vi "Arm_Graphic.vi"(10 "Boundary":T1={"X max"=310.0, "X min"=147.0, "Z max"=148.0, "Z min"=-92.0}, 11 "Calibrated Oculus Data":T2={"head"={"orientation"={"roll"=0.0, "pitch"=0.0, "yaw"=0.0}, "position"={"x"=0.0, "y"=0.0, "z"=0.0}}, "hands"={"left"={"position"={"x"=0.0, "y"=0.0, "z"=0.0}, "orientation"={"roll"=0.0, "pitch"=0.0, "yaw"=0.0}}, "right"={"position"={"x"=290.0, "y"=70.0, "z"=7.0}, "orientation"={"roll"=0.0, "pitch"=0.0, "yaw"=0.0}}}, "buttons"={"a"=FALSE, "b"=FALSE, "x"=FALSE, "y"=FALSE, "menu"=FALSE, "leftTrig"=0.0, "rightTrig"=0.0, "leftGrip"=0.0, "rightGrip"=0.0, "left_jstick"={"x"=0.0, "y"=0.0, "button"=FALSE}, "right_jstick"={"x"=0.0, "y"=0.0, "button"=FALSE}}}) -> (3 "Scene Display":refnum<vi>(3d-picture))   [LabVIEW 2017]
uses:
  Calibrated Oculus Data.ctl
  <vilib>/Utility/miscctls.llb/LVRectTypeDef.ctl
  <vilib>/picture/3D Picture Control/Object/Create Object (drawable).vi
  <vilib>/picture/3D Picture Control/Object/Create Object (name).vi
  <vilib>/picture/3D Picture Control/Object/Add Object (reference).vi
  <vilib>/express/express arith-compare/Formula/XNode/ExpressFormulaBlockNode.xnode
  <vilib>/picture/3D Picture Control/NI_3D Picture Control.lvlib
panel:
  in  "Axis label?":bool=TRUE
  out "Phi1":dbl=1.0525167643137534
  in  "R2":sgl=158.8
  in  "R1":sgl=142.0
  out "R3'":dbl=260.2363744396104
  out "r3 |x,y|":dbl=298.328677803526
  out "Theta1":sgl=1.0769706
  out "Omega":sgl=0.23684876
  in  "Up Direction":cluster{"X":sgl, "Y":sgl, "Z":sgl}={"X"=0.0, "Y"=1.0, "Z"=0.0}
  in  "Target":cluster{"X":sgl, "Y":sgl, "Z":sgl}={"X"=100.0, "Y"=100.0, "Z"=0.0}
  in  "Camera Position":cluster{"X":sgl, "Y":sgl, "Z":sgl}={"X"=300.0, "Y"=400.0, "Z"=400.0}
  in  "Rendering Destination":enum16{"Scene Window", "Scene Display"}(ring)=enum."Scene Display"
  in  "Camera Controller":enum16{"None", "Spherical", "Flying"}(ring)=enum."Spherical"
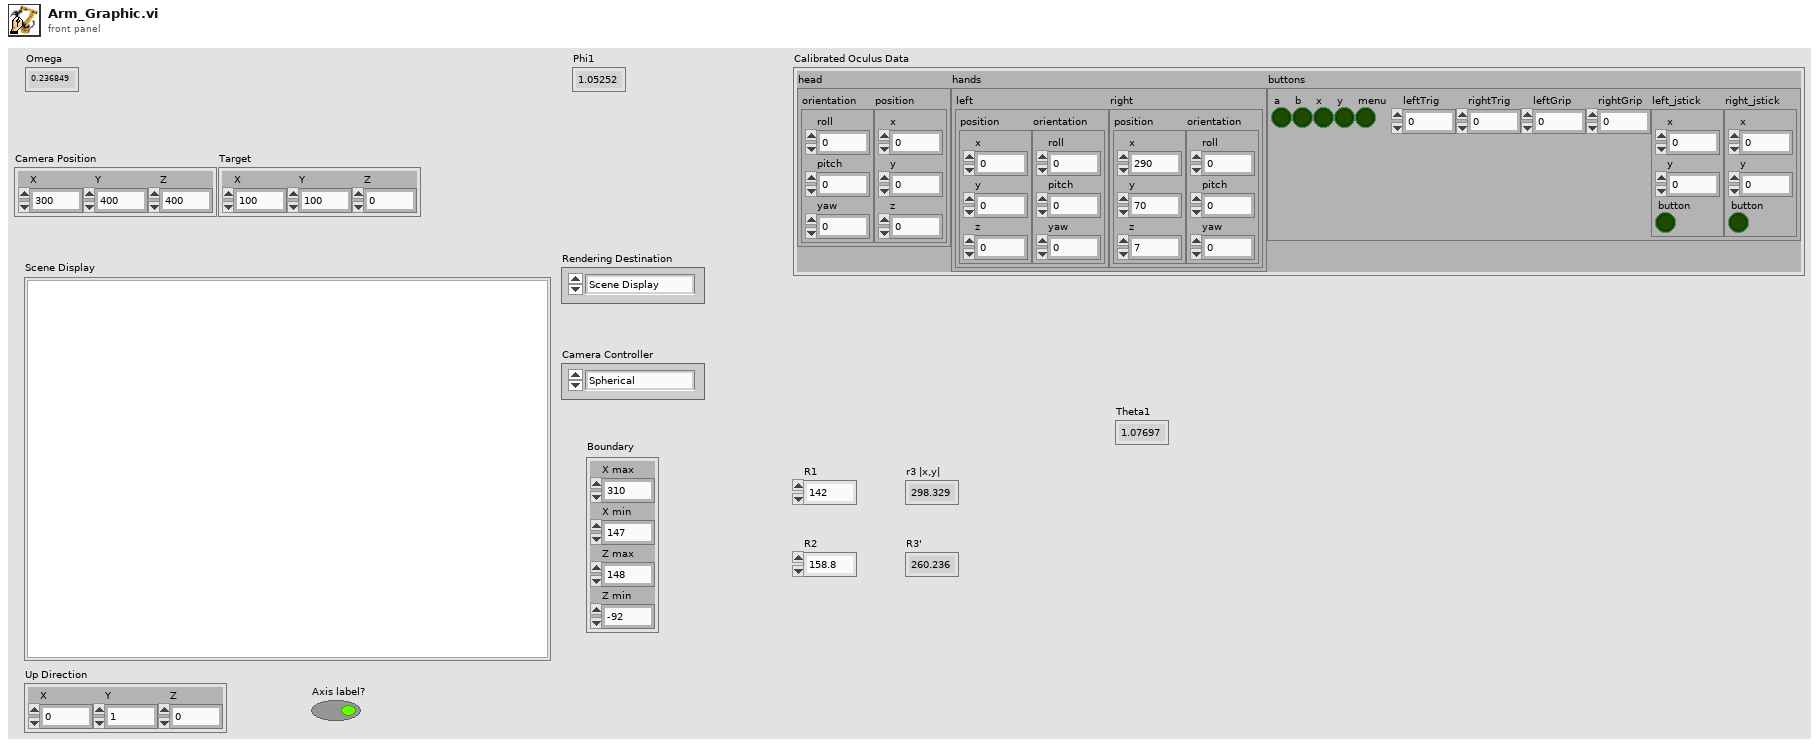
[diagram p1: front panel]
types:
  T1 = cluster{"X max":dbl, "X min":dbl, "Z max":dbl, "Z min":dbl}
  T2 = typedef "Calibrated Oculus Data.ctl" = cluster{"head":cluster{"orientation":cluster{"roll":dbl, "pitch":dbl, "yaw":dbl}, "position":cluster{"x":dbl, "y":dbl, "z":dbl}}, "hands":cluster{"left":cluster{"position":cluster{"x":dbl, "y":dbl, "z":dbl}, "orientation":cluster{"roll":dbl, "pitch":dbl, "yaw":dbl}}, "right":cluster{"position":cluster{"x":dbl, "y":dbl, "z":dbl}, "orientation":cluster{"roll":dbl, "pitch":dbl, "yaw":dbl}}}, "buttons":cluster{"a":bool, "b":bool, "x":bool, "y":bool, "menu":bool, "leftTrig":dbl, "rightTrig":dbl, "leftGrip":dbl, "rightGrip":dbl, "left_jstick":cluster{"x":dbl, "y":dbl, "button":bool}, "right_jstick":cluster{"x":dbl, "y":dbl, "button":bool}}}
  T3 = cluster{"Red":sgl, "Green":sgl, "Blue":sgl, "Alpha":sgl}
  T4 = cluster{"head":cluster{"orientation":cluster{"roll":dbl, "pitch":dbl, "yaw":dbl}, "position":cluster{"x":dbl, "y":dbl, "z":dbl}}, "hands":cluster{"left":cluster{"position":cluster{"x":dbl, "y":dbl, "z":dbl}, "orientation":cluster{"roll":dbl, "pitch":dbl, "yaw":dbl}}, "right":cluster{"position":cluster{"x":dbl, "y":dbl, "z":dbl}, "orientation":cluster{"roll":dbl, "pitch":dbl, "yaw":dbl}}}, "buttons":cluster{"a":bool, "b":bool, "x":bool, "y":bool, "menu":bool, "leftTrig":dbl, "rightTrig":dbl, "leftGrip":dbl, "rightGrip":dbl, "left_jstick":cluster{"x":dbl, "y":dbl, "button":bool}, "right_jstick":cluster{"x":dbl, "y":dbl, "button":bool}}}
  T5 = enum16{"Open", "Minimized", "Maximized", "Hidden"}
  T6 = typedef "LVRectTypeDef.ctl" = cluster{"Left":i16, "Top":i16, "Right":i16, "Bottom":i16}
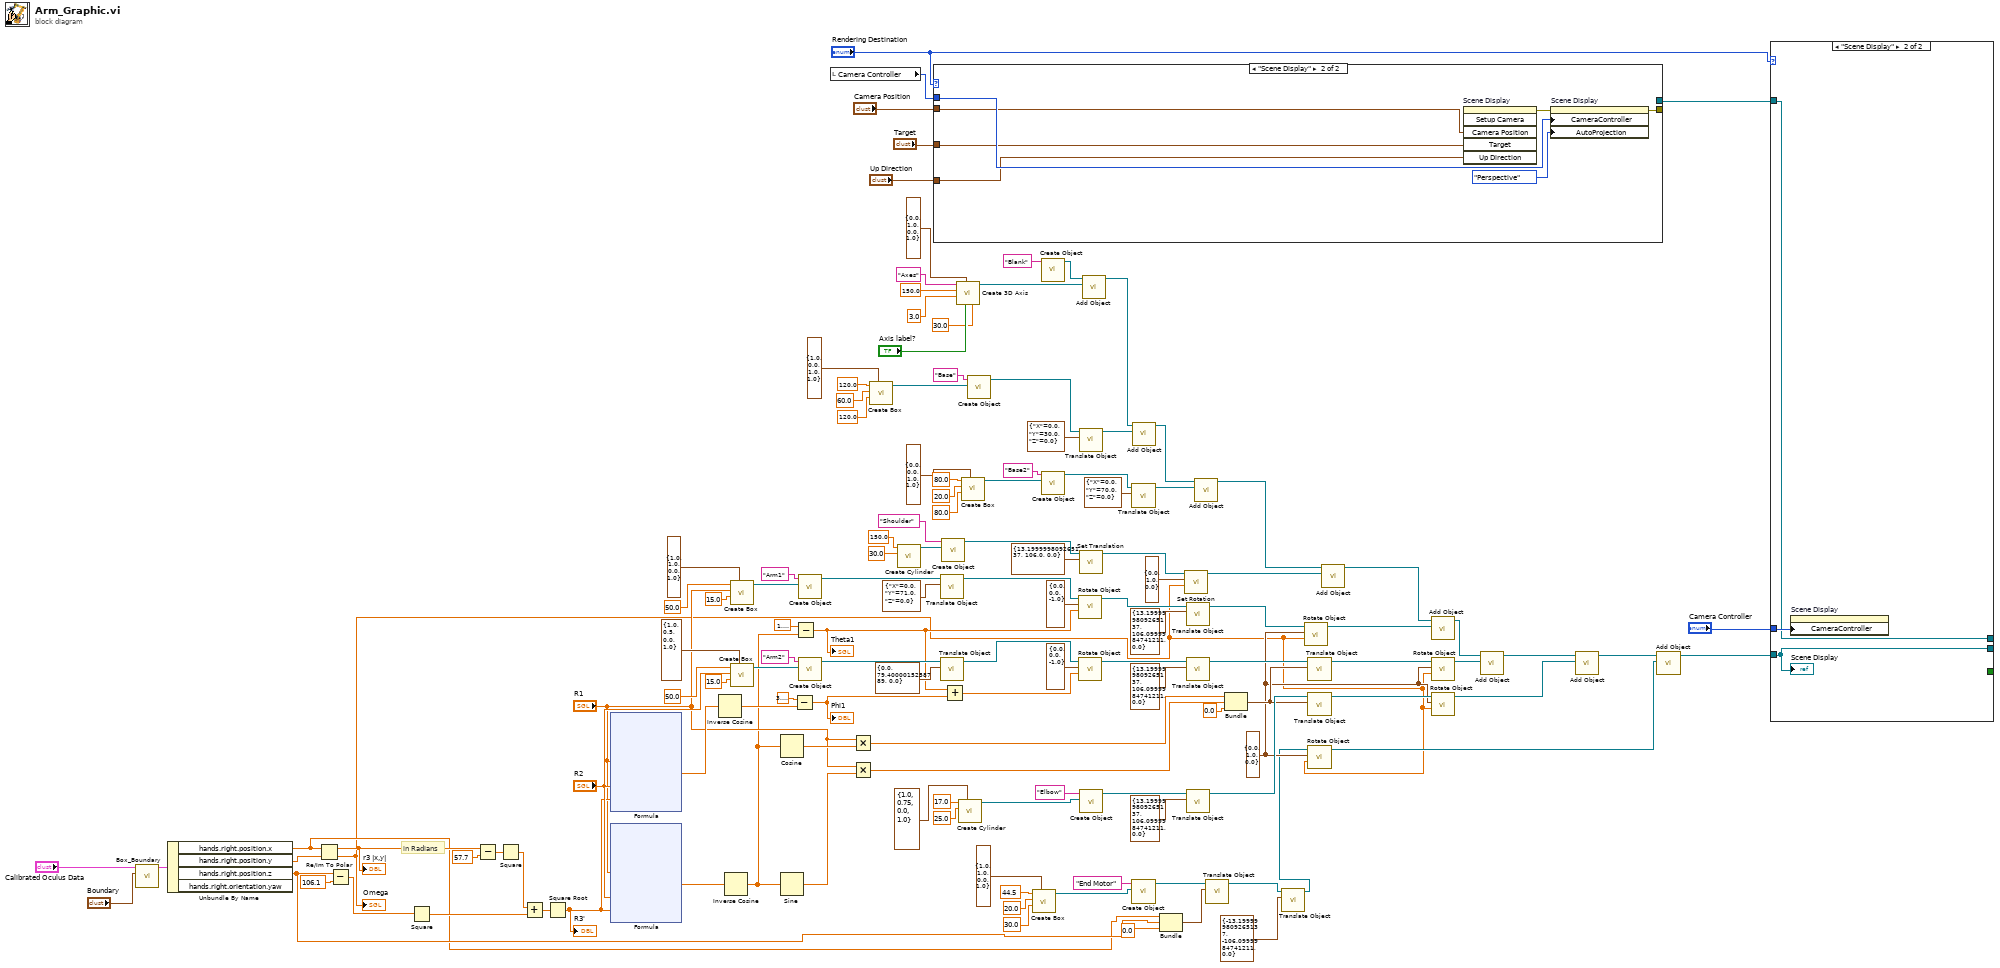
[diagram p0: block diagram]
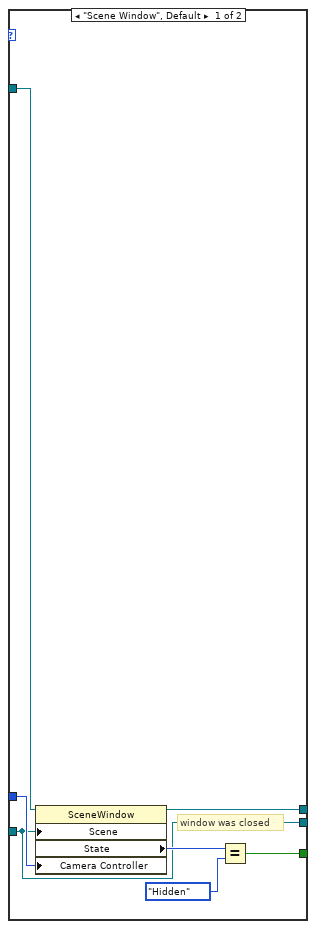
[diagram p2: hidden frame]
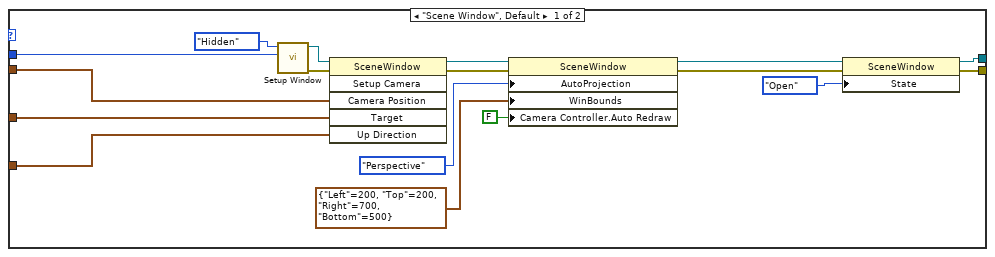
[diagram p3: hidden frame]
diagram:
  w9 = cluster{"X":sgl, "Y":sgl, "Z":sgl} {"X"=0.0, "Y"=1.0, "Z"=0.0} ("Axis")
  # "in Radians"
  n1 = call "Box_Boundary.vi"("Boundary"="Boundary", "Oculus Data in"="Calibrated Oculus Data") -> ("Oculus Data out"=w22:T4)  [unwired: 8 in, 1 out]
  n2 = Unbundle By Name(w22) -> ("hands.right.position.x"=w5:dbl, "hands.right.position.y"=w88:dbl, "hands.right.position.z"=w6:dbl)  [unwired: 1 out]
  n3 = Re/Im To Polar(2:w88, 3:w5) -> (0:w1:dbl, 1:w79:dbl)
  "Omega" <- w1
  "r3 |x,y|" <- w79
  n4 = Subtract(x=w6, y=106.1) -> (x-y=w76:dbl)
  n5 = Square(x=w76) -> (x^2=w74:dbl)
  n6 = Subtract(x=w79, y=57.7) -> (x-y=w77:dbl)
  n7 = Square(x=w77) -> (x^2=w75:dbl)
  n8 = Add(x=w75, y=w74) -> (x+y=w73:dbl)
  n9 = Square Root(x=w73) -> (sqrt(x)=w51:dbl)
  "R3'" <- w51
  n10 = xnode "Formula"("R1"="R1", "R2"="R2", "R3"=w51) -> ("Result"=w53:dbl)  [unwired: 1 in, 1 out]
  n11 = xnode "Formula"("R1"="R1", "R2"="R2", "R3"=w51) -> ("Result"=w72:dbl)  [unwired: 1 in, 1 out]
  n12 = Inverse Cosine(1:w53) -> (0:w49:dbl)
  n13 = Inverse Cosine(1:w72) -> (0:w37:dbl)
  n14 = call <vilib>:"Create Box.vi"("Color"=T3 {"Red"=1.0, "Green"=1.0, "Blue"=0.0, "Alpha"=1.0}, "Length Z"=sgl 15.0, "Length Y"="R1", "Length X"=sgl 50.0) -> ("New Box Refnum"=w133:refnum<vi>)  [unwired: 6 in, 1 out]
  n15 = call <vilib>:"Create Box.vi"("Color"=T3 {"Red"=1.0, "Green"=0.5, "Blue"=0.0, "Alpha"=1.0}, "Length Z"=sgl 15.0, "Length Y"="R2", "Length X"=sgl 50.0) -> ("New Box Refnum"=w101:refnum<vi>)  [unwired: 6 in, 1 out]
  n16 = Cosine(x=w37) -> (cos(x)=w40:dbl)
  n17 = Sine(x=w37) -> (sin(x)=w39:dbl)
  n18 = Subtract(x=3.141592653589793, y=w49) -> (x-y=w48:dbl)
  "Phi1" <- w48
  n19 = Subtract(x=1.5707963267948966, y=w37) -> (x-y=w47:dbl)
  "Theta1" <- w47
  n20 = call-poly <vilib>:"Create Object.vi"("Geometry"=w133, "Name"="Arm1") -> ("Scene:New Object"=w63:refnum<vi>)  [unwired: 8 in, 1 out]
  n21 = call-poly <vilib>:"Create Object.vi"("Geometry"=w101, "Name"="Arm2") -> ("Scene:New Object"=w55:refnum<vi>)  [unwired: 8 in, 1 out]
  n22 = local read "Camera Controller"() -> (w130:enum16{"None", "Spherical", "Flying"})
  n23 = Multiply(x="R1", y=w40) -> (x*y=w36:dbl)
  n24 = Multiply(x="R1", y=w39) -> (x*y=w35:dbl)
  n25 = call <vilib>:"Create Box.vi"("Color"=T3 {"Red"=1.0, "Green"=0.0, "Blue"=1.0, "Alpha"=1.0}, "Length Z"=sgl 120.0, "Length Y"=sgl 60.0, "Length X"=sgl 120.0) -> ("New Box Refnum"=w131:refnum<vi>)  [unwired: 6 in, 1 out]
  n26 = call <vilib>:"Create Cylinder.vi"("Radius"=sgl 30.0 ("Length Y"), "Height"=sgl 150.0 ("Length X")) -> ("New Cylinder Refnum"=w122:refnum<vi>)  [unwired: 8 in, 1 out]
  n27 = case shown="\"Scene Display\"" "Rendering Destination" {
    tunnel: w130 -> [w143 w157]
    tunnel: "Camera Position" -> [w145 w156]
    tunnel: "Target" -> [w146 w155]
    tunnel: "Up Direction" -> [w147 w154]
    tunnel: [w140 _] -> w87
    tunnel: [w136 w153] -> _
    frame "Scene Window", Default {
      n28 = call <vilib>:"Setup Window.vi"("Camera Controller"=w143, "Window State"=T5."Hidden") -> ("error out"=w139:errorcluster, "New Window Refnum"=w149:refnum<vi>)  [unwired: 1 in, 7 out]
      n29 = invoke class="SceneWindow" method="Setup Camera"(reference=w149, error in=w139, "Camera Position"=w145, "Target"=w146, "Up Direction"=w147) -> (reference out=w148:refnum<vi>, error out=w138:errorcluster)  [unwired: 1 in, 4 out]
      n30 = property class="SceneWindow"(reference=w148, error in=w138, "AutoProjection"=enum16{"None", "Perspective", "Orthographic"}."Perspective" ("Automatic Projection Mode"), "WinBounds"=T6 {"Left"=200, "Top"=200, "Right"=700, "Bottom"=500} ("Window Bounds"), "Camera Controller.Auto Redraw"=FALSE ("Camera Controller:Auto Redraw")) -> (reference out=w141:refnum<vi>, error out=w137:errorcluster)
      n31 = property class="SceneWindow"(reference=w141, error in=w137, "State"=T5."Open" ("Window State")) -> (reference out=w140:refnum<vi>, error out=w136:errorcluster)
    }
    frame "Scene Display" {
      n32 = invoke on="Scene Display" class="SceneGraphDisp (strict)" method="Setup Camera"("Camera Position"=w156, "Target"=w155, "Up Direction"=w154) -> (error out=w158:errorcluster)  [unwired: 3 in, 5 out]
      n33 = property on="Scene Display" class="SceneGraphDisp (strict)"(error in=w158, "CameraController"=w157, "AutoProjection"=enum16{"None", "Perspective", "Orthographic"}."Perspective" ("Auto Projection Mode")) -> (error out=w153:errorcluster)  [unwired: 1 in, 1 out]
    }
  }
  n34 = call <vilib>:"Translate Object.vi"("Translation"=cluster{"X":sgl, "Y":sgl, "Z":sgl} {"X"=0.0, "Y"=71.0, "Z"=0.0}, "Scene.Object In"=w63) -> ("Scene.Object Out"=w65:refnum<vi>)  [unwired: 1 in, 8 out]
  n35 = call <vilib>:"Translate Object.vi"("Translation"=cluster{"X":sgl, "Y":sgl, "Z":sgl} {"X"=0.0, "Y"=79.4, "Z"=0.0}, "Scene.Object In"=w55) -> ("Scene.Object Out"=w58:refnum<vi>)  [unwired: 1 in, 8 out]
  n36 = call-poly <vilib>:"Create Object.vi"("Geometry"=w122, "Name"="Shoulder") -> ("Scene:New Object"=w83:refnum<vi>)  [unwired: 8 in, 1 out]
  n37 = Add(x=w47, y=w48) -> (x+y=w46:dbl)
  n38 = call <vilib>:"Create 3D Axis.vi"("Character Size"=sgl 30.0, "Axis label?"="Axis label?", "Color"=T3 {"Red"=0.0, "Green"=1.0, "Blue"=0.0, "Alpha"=1.0}, "Radius"=sgl 3.0, "Length"=sgl 150.0, "Name"="Axes") -> ("New Object Refnum"=w97:refnum<vi>)  [unwired: 4 in, 1 out]
  n39 = call <vilib>:"Create Cylinder.vi"("Color"=T3 {"Red"=1.0, "Green"=0.75, "Blue"=0.0, "Alpha"=1.0}, "Radius"=sgl 25.0 ("Length Y"), "Height"=sgl 17.0 ("Length X")) -> ("New Cylinder Refnum"=w33:refnum<vi>)  [unwired: 7 in, 1 out]
  n40 = call <vilib>:"Create Box.vi"("Color"=T3 {"Red"=0.0, "Green"=0.0, "Blue"=1.0, "Alpha"=1.0}, "Length Z"=sgl 80.0, "Length Y"=sgl 20.0, "Length X"=sgl 80.0) -> ("New Box Refnum"=w112:refnum<vi>)  [unwired: 6 in, 1 out]
  n41 = call-poly <vilib>:"Create Object.vi"("Geometry"=w131, "Name"="Base") -> ("Scene:New Object"=w89:refnum<vi>)  [unwired: 8 in, 1 out]
  n42 = call <vilib>:"Create Box.vi"("Color"=T3 {"Red"=1.0, "Green"=1.0, "Blue"=0.0, "Alpha"=1.0}, "Length Z"=sgl 30.0, "Length Y"=sgl 20.0, "Length X"=sgl 44.5) -> ("New Box Refnum"=w16:refnum<vi>)  [unwired: 6 in, 1 out]
  n43 = call-poly <vilib>:"Create Object.vi"("Name"="Blank") -> ("Scene:New Object"=w98:refnum<vi>)  [unwired: 9 in, 1 out]
  n44 = call-poly <vilib>:"Create Object.vi"("Geometry"=w112, "Name"="Base2") -> ("Scene:New Object"=w92:refnum<vi>)  [unwired: 8 in, 1 out]
  n45 = call <vilib>:"Rotate Object.vi"("Angle"=w47, "Axis"=cluster{"X":sgl, "Y":sgl, "Z":sgl} {"X"=0.0, "Y"=0.0, "Z"=-1.0}, "Scene.Object In"=w65) -> ("Scene.Object Out"=w68:refnum<vi>)  [unwired: 7 in, 1 out]
  n46 = call <vilib>:"Rotate Object.vi"("Angle"=w46, "Axis"=cluster{"X":sgl, "Y":sgl, "Z":sgl} {"X"=0.0, "Y"=0.0, "Z"=-1.0}, "Scene.Object In"=w58) -> ("Scene.Object Out"=w60:refnum<vi>)  [unwired: 7 in, 1 out]
  n47 = call <vilib>:"Translate Object.vi"("Translation"=cluster{"X":sgl, "Y":sgl, "Z":sgl} {"X"=0.0, "Y"=30.0, "Z"=0.0}, "Scene.Object In"=w89) -> ("Scene.Object Out"=w90:refnum<vi>)  [unwired: 1 in, 8 out]
  n48 = call <vilib>:"Set Translation.vi"("Translation"=cluster{"X":sgl, "Y":sgl, "Z":sgl} {"X"=13.2, "Y"=106.0, "Z"=0.0}, "Scene Object"=w83) -> ("Translated Object"=w85:refnum<vi>)  [unwired: 8 in, 1 out]
  n49 = call-poly <vilib>:"Create Object.vi"("Geometry"=w33, "Name"="Elbow") -> ("Scene:New Object"=w29:refnum<vi>)  [unwired: 8 in, 1 out]
  n50 = call-poly <vilib>:"Add Object.vi"("New Object In"=w97, "Scene Object In"=w98) -> ("Scene Object Out"=w96:refnum<vi>)  [unwired: 7 in, 2 out]
  n51 = call <vilib>:"Translate Object.vi"("Translation"=cluster{"X":sgl, "Y":sgl, "Z":sgl} {"X"=0.0, "Y"=70.0, "Z"=0.0}, "Scene.Object In"=w92) -> ("Scene.Object Out"=w93:refnum<vi>)  [unwired: 1 in, 8 out]
  n52 = call-poly <vilib>:"Create Object.vi"("Geometry"=w16, "Name"="End Motor") -> ("Scene:New Object"=w11:refnum<vi>)  [unwired: 8 in, 1 out]
  n53 = call-poly <vilib>:"Add Object.vi"("New Object In"=w90, "Scene Object In"=w96) -> ("Scene Object Out"=w106:refnum<vi>)  [unwired: 7 in, 2 out]
  n54 = Bundle("x"=w5, "z"=w6, "X"=sgl 0.0) -> (w8:cluster{"x":dbl, "z":dbl, "X":sgl})  [unwired: 1 in]
  n55 = call <vilib>:"Set Rotation.vi"("Angle"=w1, "Axis"=cluster{"X":sgl, "Y":sgl, "Z":sgl} {"X"=0.0, "Y"=1.0, "Z"=0.0}, "Scene Object"=w85) -> ("Rotated Scene Object"=w82:refnum<vi>)  [unwired: 7 in, 1 out]
  n56 = call <vilib>:"Translate Object.vi"("Translation"=cluster{"X":sgl, "Y":sgl, "Z":sgl} {"X"=13.2, "Y"=106.1, "Z"=0.0}, "Scene.Object In"=w68) -> ("Scene.Object Out"=w70:refnum<vi>)  [unwired: 1 in, 8 out]
  n57 = call <vilib>:"Translate Object.vi"("Translation"=cluster{"X":sgl, "Y":sgl, "Z":sgl} {"X"=13.2, "Y"=106.1, "Z"=0.0}, "Scene.Object In"=w60) -> ("Scene.Object Out"=w43:refnum<vi>)  [unwired: 1 in, 8 out]
  n58 = call <vilib>:"Translate Object.vi"("Translation"=cluster{"X":sgl, "Y":sgl, "Z":sgl} {"X"=13.2, "Y"=106.1, "Z"=0.0}, "Scene.Object In"=w29) -> ("Scene.Object Out"=w26:refnum<vi>)  [unwired: 1 in, 8 out]
  n59 = call-poly <vilib>:"Add Object.vi"("New Object In"=w93, "Scene Object In"=w106) -> ("Scene Object Out"=w105:refnum<vi>)  [unwired: 7 in, 2 out]
  n60 = call <vilib>:"Translate Object.vi"("Translation"=w8, "Scene.Object In"=w11) -> ("Scene.Object Out"=w3:refnum<vi>)  [unwired: 1 in, 8 out]
  n61 = Bundle(w36, w35, "X"=sgl 0.0) -> (w25:cluster{dbl, dbl, "X":sgl})  [unwired: 1 in]
  n62 = call <vilib>:"Translate Object.vi"("Translation"=cluster{"X":sgl, "Y":sgl, "Z":sgl} {"X"=-13.2, "Y"=-106.1, "Z"=0.0}, "Scene.Object In"=w3) -> ("Scene.Object Out"=w4:refnum<vi>)  [unwired: 1 in, 8 out]
  n63 = call <vilib>:"Rotate Object.vi"("Angle"=w1, "Axis"=w9, "Scene.Object In"=w70) -> ("Scene.Object Out"=w69:refnum<vi>)  [unwired: 7 in, 1 out]
  n64 = call <vilib>:"Translate Object.vi"("Translation"=w25, "Scene.Object In"=w43) -> ("Scene.Object Out"=w44:refnum<vi>)  [unwired: 1 in, 8 out]
  n65 = call <vilib>:"Translate Object.vi"("Translation"=w25, "Scene.Object In"=w26) -> ("Scene.Object Out"=w24:refnum<vi>)  [unwired: 1 in, 8 out]
  n66 = call <vilib>:"Rotate Object.vi"("Angle"=w1, "Axis"=w9, "Scene.Object In"=w4) -> ("Scene.Object Out"=w10:refnum<vi>)  [unwired: 7 in, 1 out]
  n67 = call-poly <vilib>:"Add Object.vi"("New Object In"=w82, "Scene Object In"=w105) -> ("Scene Object Out"=w99:refnum<vi>)  [unwired: 7 in, 2 out]
  n68 = call-poly <vilib>:"Add Object.vi"("New Object In"=w69, "Scene Object In"=w99) -> ("Scene Object Out"=w95:refnum<vi>)  [unwired: 7 in, 2 out]
  n69 = call <vilib>:"Rotate Object.vi"("Angle"=w1, "Axis"=w9, "Scene.Object In"=w44) -> ("Scene.Object Out"=w56:refnum<vi>)  [unwired: 7 in, 1 out]
  n70 = call <vilib>:"Rotate Object.vi"("Angle"=w1, "Axis"=w9, "Scene.Object In"=w24) -> ("Scene.Object Out"=w23:refnum<vi>)  [unwired: 7 in, 1 out]
  n71 = call-poly <vilib>:"Add Object.vi"("New Object In"=w56, "Scene Object In"=w95) -> ("Scene Object Out"=w30:refnum<vi>)  [unwired: 7 in, 2 out]
  n72 = call-poly <vilib>:"Add Object.vi"("New Object In"=w23, "Scene Object In"=w30) -> ("Scene Object Out"=w19:refnum<vi>)  [unwired: 7 in, 2 out]
  n73 = call-poly <vilib>:"Add Object.vi"("New Object In"=w10, "Scene Object In"=w19) -> ("Scene Object Out"=w18:refnum<vi>)  [unwired: 7 in, 2 out]
  n74 = case shown="\"Scene Display\"" "Rendering Destination" {
    tunnel: w87 -> [w166 w167]
    tunnel: w18 -> [w161 w168]
    tunnel: [w163 _] -> _
    tunnel: "Camera Controller" -> [w162 w169]
    tunnel: [w161 w168] -> _
    tunnel: [w160 w167] -> _
    frame "Scene Window", Default {
      # "window was closed"
      n75 = property class="SceneWindow"(reference=w166, "Scene"=w161, "Camera Controller"=w162) -> (reference out=w160:refnum<vi>, "State"=w165:T5)  [unwired: 1 in, 1 out]
      n76 = Equal?(x=w165, y=T5."Hidden" ("Window State")) -> (x = y?=w163:bool)
    }
    frame "Scene Display" {
      n77 = property on="Scene Display" class="SceneGraphDisp (strict)"("CameraController"=w169) -> ()  [unwired: 2 in, 2 out]
      "Scene Display" <- w168
    }
  }
